vi "String to Tree Inner Part.vi"(4 "structure before":T2(array[cluster]), 5 "dummy":T1, 6 "error situation before":i32, 7 "dot or comma":string) -> (0 "error in formula-write":string, 1 "structure after":T2(array[cluster]), 2 "error situation after":i32, 3 "end of analysis":bool)   [LabVIEW 2009]
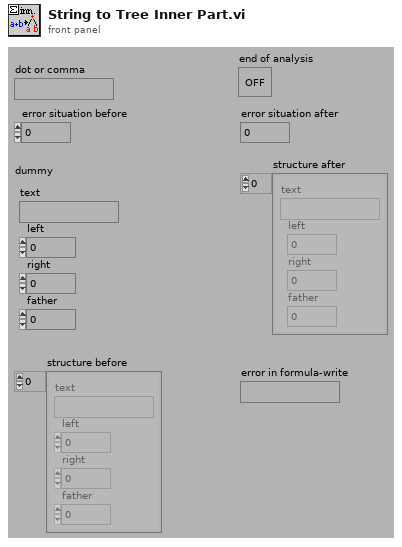
[diagram p1: front panel]
types:
  T1 = cluster{"text":string, "left":i32, "right":i32, "father":i32}
  T2 = cluster{"text":string, "left":i32, "right":i32, "father":i32}[]
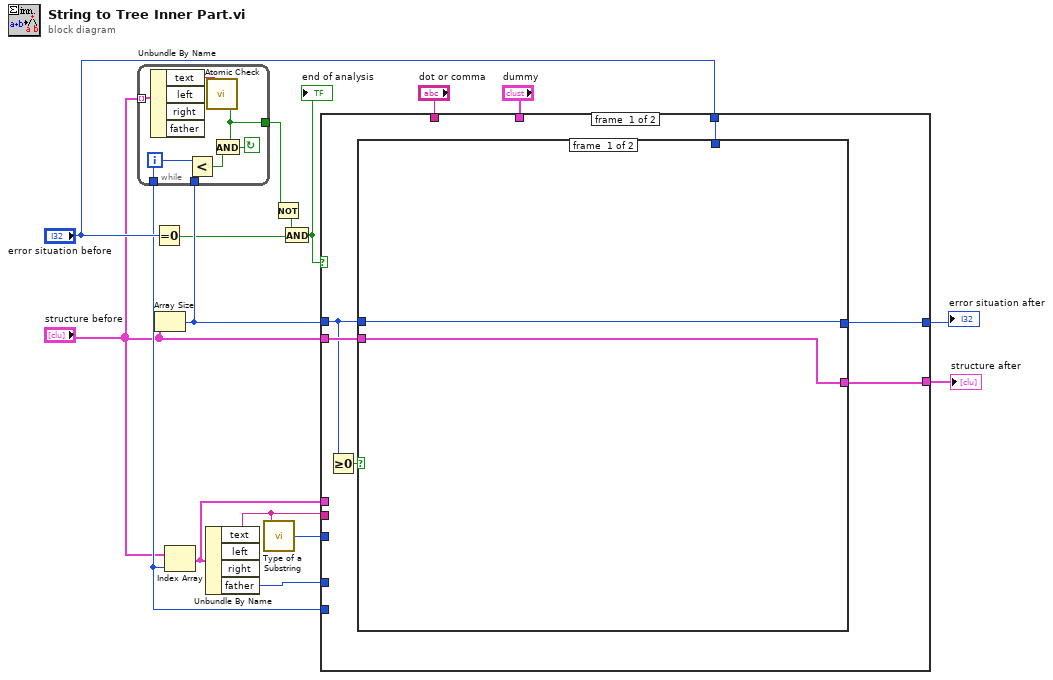
[diagram p0: block diagram]
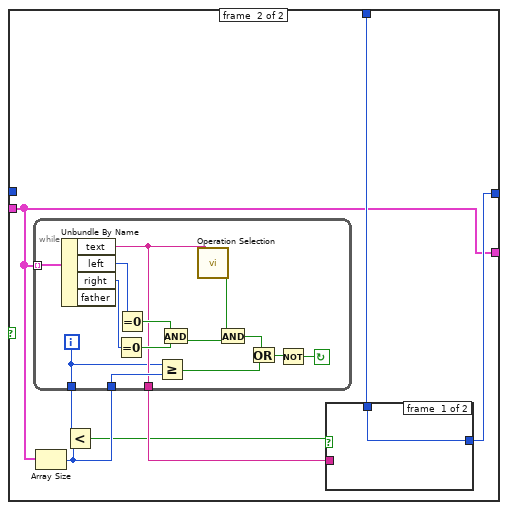
[diagram p2: hidden frame]
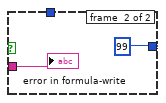
[diagram p3: hidden frame]
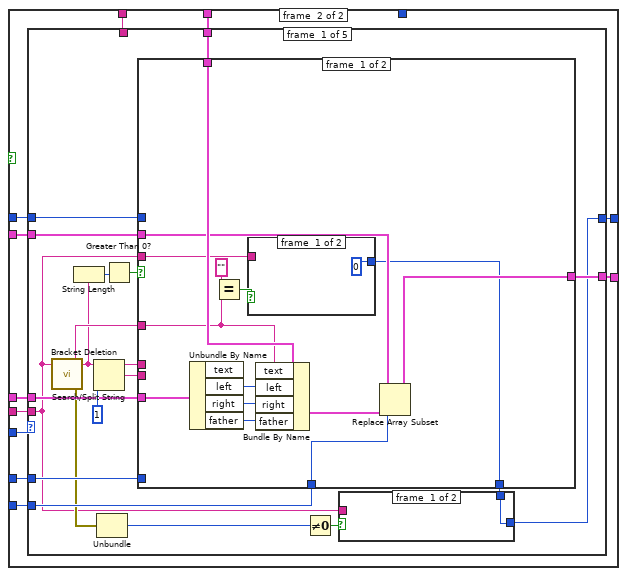
[diagram p4: hidden frame]
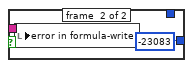
[diagram p5: hidden frame]
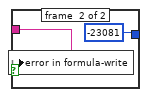
[diagram p6: hidden frame]
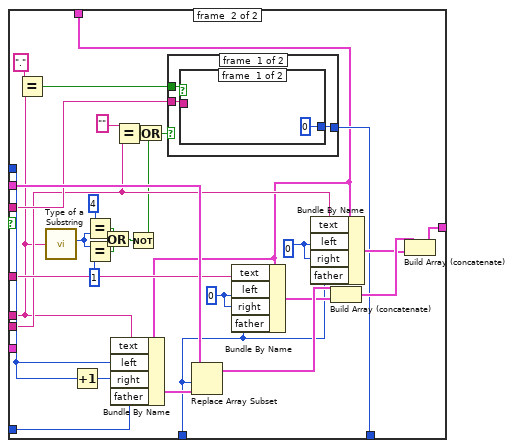
[diagram p7: hidden frame]
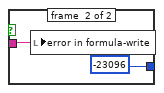
[diagram p8: hidden frame]
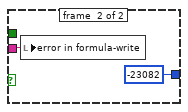
[diagram p9: hidden frame]
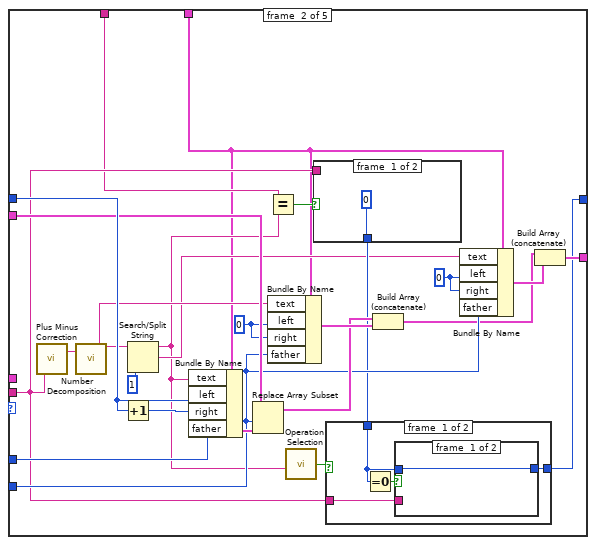
[diagram p10: hidden frame]
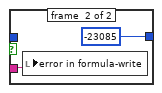
[diagram p11: hidden frame]
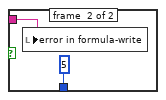
[diagram p13: hidden frame]
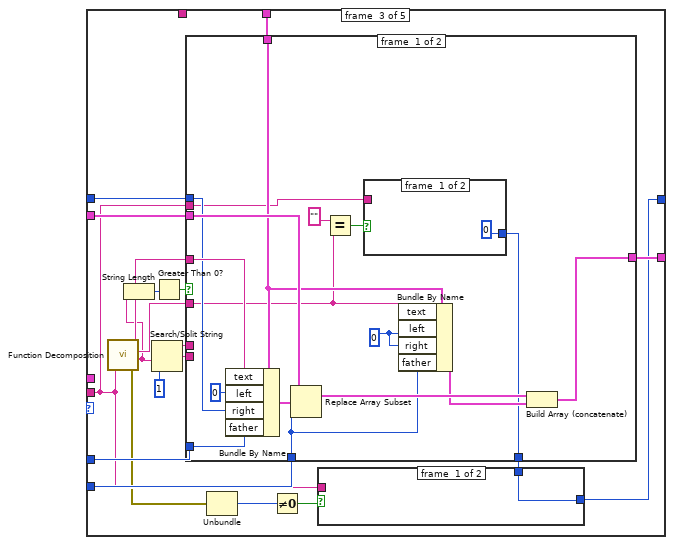
[diagram p14: hidden frame]
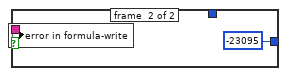
[diagram p15: hidden frame]
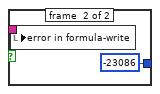
[diagram p16: hidden frame]
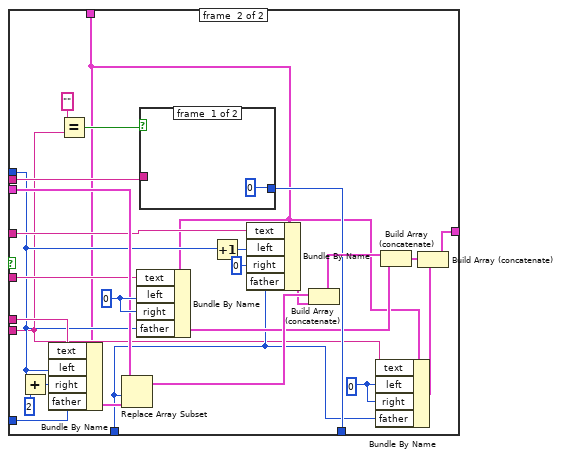
[diagram p17: hidden frame]
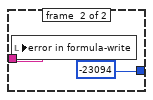
[diagram p18: hidden frame]
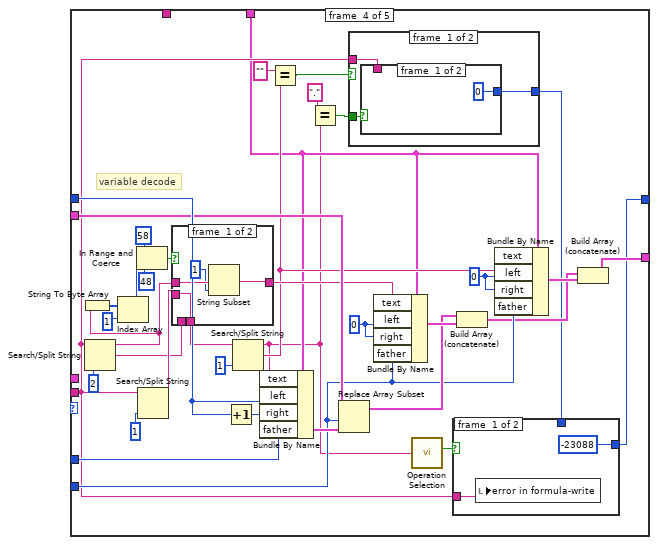
[diagram p19: hidden frame]
diagram:
  n1 = Equal To 0?(x="error situation before") -> (x = 0?=w4:bool)
  n2 = Array Size(array="structure before") -> (size(s)=w7:i32)
  n3 = while {
    tunnel: [w19] -> w8
    tunnel: w7 -> [w21]
    tunnel: [w17] -> w6
    tunnel: "structure before" -> [w23] mode=indexing
    i -> [w17]
    stop <- w18 continue-if-true
    n4 = Unbundle By Name(w23) -> ("text"=w22:string)  [unwired: 3 out]
    n5 = Less?(x=w17, y=w21) -> (x < y?=w20:bool)
    n6 = call "Atomic Check.VI"("string"=w22) -> ("atomic"=w19:bool)
    n7 = And(x=w19, y=w20) -> (x .and. y?=w18:bool)
  }
  n8 = Index Array(array="structure before", index=w6) -> (element=w9:T1)
  n9 = Unbundle By Name(w9) -> ("text"=w12:string, "father"=w5:i32)  [unwired: 2 out]
  n10 = call "Type of a Substring.VI"("item"=w12) -> ("type"=w14:i32)
  n11 = Not(x=w8) -> (.not. x?=w3:bool)
  n12 = And(x=w3, y=w4) -> (x .and. y?=w13:bool)
  "end of analysis" <- w13
  n13 = case shown="True" w13 {
    tunnel: w7 -> [w24 w66]
    tunnel: [w26 w65] -> w16
    tunnel: "structure before" -> [w29 w64]
    tunnel: w6 -> [_ w63]
    tunnel: w5 -> [_ w62]
    tunnel: w12 -> [_ w61]
    tunnel: w14 -> [_ w60]
    tunnel: w9 -> [_ w59]
    tunnel: [w28 w58] -> w10
    tunnel: "error situation before" -> [w27 _]
    tunnel: "dot or comma" -> [_ w57]
    tunnel: "dummy" -> [_ w56]
    frame #0 {
      n14 = Greater Or Equal To 0?(x=w24) -> (x >= 0?=w25:bool)
      n15 = case shown="True" w25 {
        tunnel: w27 -> [_ w36]
        tunnel: [w30 w35] -> w28
        tunnel: w29 -> [w31 w32]
        tunnel: [w31 w32] -> w26
        tunnel: w24 -> [w30 _]
        frame #0 {
        }
        frame #1 {
          n16 = Array Size(array=w32) -> (size(s)=w38:i32)
          n17 = while {
            tunnel: w38 -> [w45]
            tunnel: [w41] -> w37
            tunnel: [w39] -> w33
            tunnel: w32 -> [w52] mode=indexing
            i -> [w39]
            stop <- w46 continue-if-true
            n18 = Unbundle By Name(w52) -> ("text"=w41:string, "left"=w51:i32, "right"=w50:i32)  [unwired: 1 out]
            n19 = Equal To 0?(x=w50) -> (x = 0?=w48:bool)
            n20 = Equal To 0?(x=w51) -> (x = 0?=w49:bool)
            n21 = Greater Or Equal?(x=w39, y=w45) -> (x >= y?=w44:bool)
            n22 = And(x=w49, y=w48) -> (x .and. y?=w47:bool)
            n23 = call "Operation Selection.VI"("selector"=w41) -> ("result"=w40:bool)
            n24 = And(x=w40, y=w47) -> (x .and. y?=w43:bool)
            n25 = Or(x=w43, y=w44) -> (x .or. y?=w42:bool)
            n26 = Not(x=w42) -> (.not. x?=w46:bool)
          }
          n27 = Less?(x=w33, y=w38) -> (x < y?=w34:bool)
          n28 = case shown="True" w34 {
            tunnel: [w53 99] -> w35
            tunnel: w36 -> [w53 _]
            tunnel: w37 -> [_ w54]
            frame #0 {
            }
            frame #1 {
              "error in formula-write" <- w54
            }
          }
        }
      }
    }
    frame #1 {
      n29 = case shown="3" w60 {
        tunnel: w61 -> [w70 w152 w190 w263 w311]
        tunnel: w62 -> [w85 w170 w201 w293 _]
        tunnel: w66 -> [w84 w169 w195 w292 _]
        tunnel: w63 -> [w81 w161 w199 w284 _]
        tunnel: w64 -> [w83 w166 w200 w289 w312]
        tunnel: [w79 w158 w193 w269 w312] -> w65
        tunnel: w59 -> [w74 _ _ _ _]
        tunnel: [w72 w153 w191 w264 -23087] -> w58
        tunnel: w57 -> [_ w147 _ _ _]
        tunnel: w56 -> [w67 w146 w183 w257 _]
        frame #0 {
          n30 = call "Bracket Deletion.vi"("string input with brackets"=w70) -> ("string output balanced"=w82:string, "string output rest"=w77:string, "error out"=w71:errorcluster)  [unwired: 1 in]
          n31 = String Length(string=w77) -> (length=w76:i32)
          n32 = Search/Split String(string=w77, offset (0)=1) -> (substring before match=w78:string, match + rest of string=w80:string)  [unwired: 1 in, 1 out]
          n33 = Unbundle(w71) -> ("code"=w69:i32)  [unwired: 2 out]
          n34 = Greater Than 0?(x=w76) -> (x > 0?=w75:bool)
          n35 = case shown="True" w75 {
            tunnel: w78 -> [_ w108]
            tunnel: [w95 w137] -> w79
            tunnel: w67 -> [w99 w107]
            tunnel: w80 -> [_ w121]
            tunnel: w81 -> [w96 w109]
            tunnel: w82 -> [w94 w122]
            tunnel: w83 -> [w98 w130]
            tunnel: w84 -> [_ w127]
            tunnel: w85 -> [_ w126]
            tunnel: w74 -> [w103 _]
            tunnel: w70 -> [w91 w123]
            tunnel: [w90 w124] -> w73
            frame #0 {
              n36 = Unbundle By Name(w103) -> ("left"=w102:i32, "right"=w101:i32, "father"=w100:i32)  [unwired: 1 out]
              n37 = Equal?(x="", y=w94) -> (x = y?=w92:bool)
              n38 = case shown="True" w92 {
                tunnel: w91 -> [_ w106]
                tunnel: [0 -23081] -> w90
                frame #0 {
                }
                frame #1 {
                  n39 = local write "error in formula-write"(w106) -> ()
                }
              }
              n40 = Bundle By Name(cluster=w99, "text"=w94, "left"=w102, "right"=w101, "father"=w100) -> (w97:T1)
              n41 = Replace Array Subset(array=w98, new element=w97, index=w96) -> (w95:T2)
            }
            frame #1 {
              w131 = 0
              w134 = 0
              n42 = Equal?(x=".", y=w108) -> (x = y?=w110:bool)
              n43 = call "Type of a Substring.VI"("item"=w108) -> ("type"=w117:i32)
              n44 = Increment(x=w127) -> (x+1=w128:i32)
              n45 = Equal?(x=4, y=w117) -> (x = y?=w116:bool)
              n46 = Equal?(x=w117, y=1) -> (x = y?=w114:bool)
              n47 = Or(x=w116, y=w114) -> (x .or. y?=w113:bool)
              n48 = Bundle By Name(cluster=w107, "text"=w108, "left"=w127, "right"=w128, "father"=w126) -> (w129:T1)
              n49 = Equal?(x="", y=w121) -> (x = y?=w115:bool)
              n50 = Not(x=w113) -> (.not. x?=w112:bool)
              n51 = Or(x=w115, y=w112) -> (x .or. y?=w119:bool)
              n52 = case shown="True" w119 {
                tunnel: [w140 -23082] -> w124
                tunnel: w123 -> [w139 w144]
                tunnel: w110 -> [w138 _]
                frame #0 {
                  n53 = case shown="True" w138 {
                    tunnel: [0 -23096] -> w140
                    tunnel: w139 -> [_ w142]
                    frame #0 {
                    }
                    frame #1 {
                      n54 = local write "error in formula-write"(w142) -> ()
                    }
                  }
                }
                frame #1 {
                  n55 = local write "error in formula-write"(w144) -> ()
                }
              }
              n56 = Replace Array Subset(array=w130, new element=w129, index=w109) -> (w133:T2)
              n57 = Bundle By Name(cluster=w107, "text"=w122, "left"=w131, "right"=w131, "father"=w109) -> (w132:T1)
              n58 = Bundle By Name(cluster=w107, "text"=w121, "left"=w134, "right"=w134, "father"=w109) -> (w135:T1)
              n59 = Build Array (concatenate)(w133, w132) -> (w136:T2)
              n60 = Build Array (concatenate)(w136, w135) -> (w137:T2)
            }
          }
          n61 = Not Equal To 0?(x=w69) -> (x != 0?=w68:bool)
          n62 = case shown="True" w68 {
            tunnel: [w87 -23083] -> w72
            tunnel: w70 -> [_ w88]
            tunnel: w73 -> [w87 _]
            frame #0 {
            }
            frame #1 {
              n63 = local write "error in formula-write"(w88) -> ()
            }
          }
        }
        frame #1 {
          w162 = 0
          w165 = 0
          n64 = call "Plus Minus Correction.vi"("string"=w152) -> ("new string"=w157:string)  [unwired: 1 out]
          n65 = call "Number Decomposition.VI"("number string"=w157) -> ("number"=w151:string, "rest"=w150:string)  [unwired: 1 in, 1 out]
          n66 = Increment(x=w169) -> (x+1=w168:i32)
          n67 = Search/Split String(string=w150, offset (0)=1) -> (substring before match=w148:string, match + rest of string=w149:string)  [unwired: 1 in, 1 out]
          n68 = Bundle By Name(cluster=w146, "text"=w148, "left"=w169, "right"=w168, "father"=w170) -> (w167:T1)
          n69 = Replace Array Subset(array=w166, new element=w167, index=w161) -> (w163:T2)
          n70 = Equal?(x=w147, y=w148) -> (x = y?=w156:bool)
          n71 = Bundle By Name(cluster=w146, "text"=w151, "left"=w165, "right"=w165, "father"=w161) -> (w164:T1)
          n72 = call "Operation Selection.VI"("selector"=w148) -> ("result"=w155:bool)
          n73 = case shown="True" w156 {
            tunnel: [0 5] -> w154
            tunnel: w152 -> [_ w181]
            frame #0 {
            }
            frame #1 {
              n74 = local write "error in formula-write"(w181) -> ()
            }
          }
          n75 = case shown="False" w155 {
            tunnel: w154 -> [w172 w179]
            tunnel: [w174 w179] -> w153
            tunnel: w152 -> [w175 _]
            frame #0 {
              n76 = Equal To 0?(x=w172) -> (x = 0?=w173:bool)
              n77 = case shown="True" w173 {
                tunnel: w175 -> [_ w178]
                tunnel: [w176 -23085] -> w174
                tunnel: w172 -> [w176 _]
                frame #0 {
                }
                frame #1 {
                  n78 = local write "error in formula-write"(w178) -> ()
                }
              }
            }
            frame #1 {
            }
          }
          n79 = Build Array (concatenate)(w163, w164) -> (w159:T2)
          n80 = Bundle By Name(cluster=w146, "text"=w149, "left"=w162, "right"=w162, "father"=w161) -> (w160:T1)
          n81 = Build Array (concatenate)(w159, w160) -> (w158:T2)
        }
        frame #2 {
          n82 = call "Function Decomposition.VI"("function string"=w190) -> ("function text"=w196:string, "function brackets"=w194:string, "rest"=w184:string, "error out"=w187:errorcluster)  [unwired: 1 in]
          n83 = String Length(string=w184) -> (length=w189:i32)
          n84 = Search/Split String(string=w184, offset (0)=1) -> (substring before match=w198:string, match + rest of string=w197:string)  [unwired: 1 in, 1 out]
          n85 = Greater Than 0?(x=w189) -> (x > 0?=w192:bool)
          n86 = case shown="False" w192 {
            tunnel: [w213 w252] -> w193
            tunnel: w194 -> [w209 w233]
            tunnel: w183 -> [w214 w226]
            tunnel: w195 -> [w212 w230]
            tunnel: w196 -> [w221 w238]
            tunnel: w197 -> [_ w227]
            tunnel: w198 -> [_ w246]
            tunnel: w199 -> [w211 w231]
            tunnel: w200 -> [w219 w242]
            tunnel: w201 -> [w222 w240]
            tunnel: w190 -> [w207 w239]
            tunnel: [w206 w235] -> w188
            frame #0 {
              w218 = 0
              n87 = Bundle By Name(cluster=w214, "text"=w221, "left"=0, "right"=w212, "father"=w222) -> (w220:T1)
              n88 = Replace Array Subset(array=w219, new element=w220, index=w211) -> (w216:T2)
              n89 = Equal?(x="", y=w209) -> (x = y?=w208:bool)
              n90 = case shown="True" w208 {
                tunnel: w207 -> [_ w225]
                tunnel: [0 -23086] -> w206
                frame #0 {
                }
                frame #1 {
                  n91 = local write "error in formula-write"(w225) -> ()
                }
              }
              n92 = Bundle By Name(cluster=w214, "text"=w209, "left"=w218, "right"=w218, "father"=w211) -> (w215:T1)
              n93 = Build Array (concatenate)(w216, w215) -> (w213:T2)
            }
            frame #1 {
              w243 = 0
              w249 = 0
              n94 = Add(x=w230, y=2) -> (x+y=w228:i32)
              n95 = Bundle By Name(cluster=w226, "text"=w246, "left"=w230, "right"=w228, "father"=w240) -> (w241:T1)
              n96 = Equal?(x="", y=w227) -> (x = y?=w237:bool)
              n97 = Replace Array Subset(array=w242, new element=w241, index=w231) -> (w244:T2)
              n98 = Bundle By Name(cluster=w226, "text"=w233, "left"=w243, "right"=w243, "father"=w230) -> (w232:T1)
              n99 = case shown="True" w237 {
                tunnel: w239 -> [_ w255]
                tunnel: [0 -23094] -> w235
                frame #0 {
                }
                frame #1 {
                  n100 = local write "error in formula-write"(w255) -> ()
                }
              }
              n101 = Increment(x=w230) -> (x+1=w248:i32)
              n102 = Bundle By Name(cluster=w226, "text"=w238, "left"=w248, "right"=0, "father"=w231) -> (w234:T1)
              n103 = Build Array (concatenate)(w244, w234) -> (w245:T2)
              n104 = Bundle By Name(cluster=w226, "text"=w227, "left"=w249, "right"=w249, "father"=w231) -> (w251:T1)
              n105 = Build Array (concatenate)(w245, w232) -> (w250:T2)
              n106 = Build Array (concatenate)(w250, w251) -> (w252:T2)
            }
          }
          n107 = Unbundle(w187) -> ("code"=w186:i32)  [unwired: 2 out]
          n108 = Not Equal To 0?(x=w186) -> (x != 0?=w185:bool)
          n109 = case shown="True" w185 {
            tunnel: [w203 -23095] -> w191
            tunnel: w190 -> [_ w204]
            tunnel: w188 -> [w203 _]
            frame #0 {
            }
            frame #1 {
              n110 = local write "error in formula-write"(w204) -> ()
            }
          }
        }
        frame #3 {
          w285 = 0
          w288 = 0
          # "variable decode"
          n111 = Search/Split String(string=w263, offset (0)=2) -> (substring before match=w274:string, match + rest of string=w262:string)  [unwired: 1 in, 1 out]
          n112 = String To Byte Array(string=w274) -> (unsigned byte array=w280:u8[])
          n113 = Index Array(array=w280, index=1) -> (element=w276:u8)
          n114 = In Range and Coerce(upper limit=58, x=w276, lower limit=48) -> (In Range?=w275:bool)  [unwired: 1 out]
          n115 = Search/Split String(string=w263, offset (0)=1) -> (match + rest of string=w271:string)  [unwired: 1 in, 2 out]
          n116 = case shown="False" w275 {
            tunnel: w262 -> [_ w310]
            tunnel: [w308 w310] -> w258
            tunnel: [w305 w309] -> w273
            tunnel: w274 -> [w307 w309]
            tunnel: w271 -> [w308 _]
            frame #0 {
              n117 = String Subset(string=w307, length (rest)=1) -> (substring=w305:string)  [unwired: 1 in]
            }
            frame #1 {
            }
          }
          n118 = Increment(x=w292) -> (x+1=w291:i32)
          n119 = Search/Split String(string=w258, offset (0)=1) -> (substring before match=w256:string, match + rest of string=w259:string)  [unwired: 1 in, 1 out]
          n120 = Bundle By Name(cluster=w257, "text"=w256, "left"=w292, "right"=w291, "father"=w293) -> (w290:T1)
          n121 = Equal?(x="", y=w259) -> (x = y?=w267:bool)
          n122 = Equal?(x=".", y=w256) -> (x = y?=w260:bool)
          n123 = Replace Array Subset(array=w289, new element=w290, index=w284) -> (w286:T2)
          n124 = case shown="True" w267 {
            tunnel: [w299 -23093] -> w265
            tunnel: w263 -> [w297 w303]
            tunnel: w260 -> [w298 _]
            frame #0 {
              n125 = case shown="True" w298 {
                tunnel: [0 -23096] -> w299
                tunnel: w297 -> [_ w301]
                frame #0 {
                }
                frame #1 {
                  n126 = local write "error in formula-write"(w301) -> ()
                }
              }
            }
            frame #1 {
              n127 = local write "error in formula-write"(w303) -> ()
            }
          }
          n128 = Bundle By Name(cluster=w257, "text"=w273, "left"=w288, "right"=w288, "father"=w284) -> (w287:T1)
          n129 = call "Operation Selection.VI"("selector"=w256) -> ("result"=w266:bool)
          n130 = case shown="False" w266 {
            tunnel: w265 -> [_ w296]
            tunnel: [-23088 w296] -> w264
            tunnel: w263 -> [w294 _]
            frame #0 {
              n131 = local write "error in formula-write"(w294) -> ()
            }
            frame #1 {
            }
          }
          n132 = Build Array (concatenate)(w286, w287) -> (w282:T2)
          n133 = Bundle By Name(cluster=w257, "text"=w259, "left"=w285, "right"=w285, "father"=w284) -> (w283:T1)
          n134 = Build Array (concatenate)(w282, w283) -> (w269:T2)
        }
        frame #4 {
          n135 = local write "error in formula-write"(w311) -> ()
        }
      }
    }
  }
  "structure after" <- w16
  "error situation after" <- w10
